vi "Get Current Temperature.vi"(8 "error in (no error)":errorcluster, 11 "HW Evaporative Cooler in":refnum<class "HW Evaporative Cooler.lvclass">) -> (0 "error out":errorcluster, 2 "Level":dbl)   [LabVIEW 2025, in "HW Evaporative Cooler.lvclass"]
doc: "This VI specifies what variable the level controller is monitoring. When called, this VI should return the current value of that variable."
uses:
  HW Evaporative Cooler.lvclass
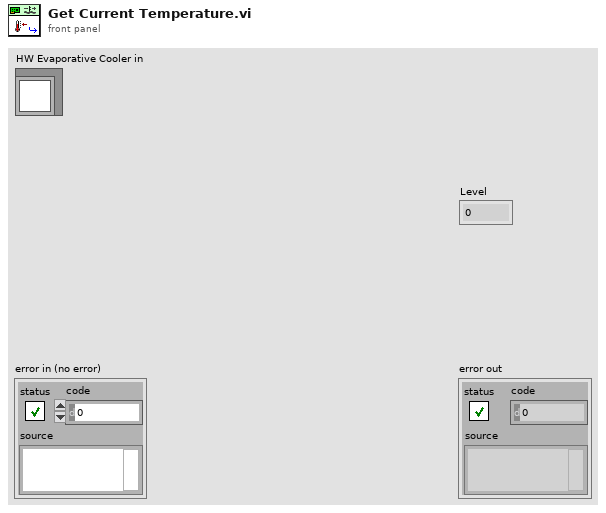
[diagram p1: front panel]
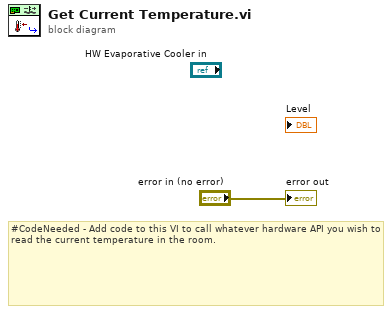
[diagram p0: block diagram]
diagram:
  # "#CodeNeeded - Add code to this VI to call whatever hardware API you wish to read the current temperature in the room."
  "error out" <- "error in (no error)"
